vi "visitCompoundGraphic.vi"(8 "error in (no error)":errorcluster, 10 "CompoundShape":refnum<class "CompoundShape.lvclass">, 11 "XMLExportVisitor in":refnum<class "XMLExportVisitor.lvclass">) -> (0 "error out":errorcluster, 2 "String":string, 3 "XMLExportVisitor out":refnum<class "XMLExportVisitor.lvclass">)   [LabVIEW 2017, in "XMLExportVisitor.lvclass"]
uses:
  XMLExportVisitor.lvclass
  CompoundShape Class/CompoundShape.lvclass
  CompoundShape Class/CompoundShape.lvclass/CompoundShape.ctl
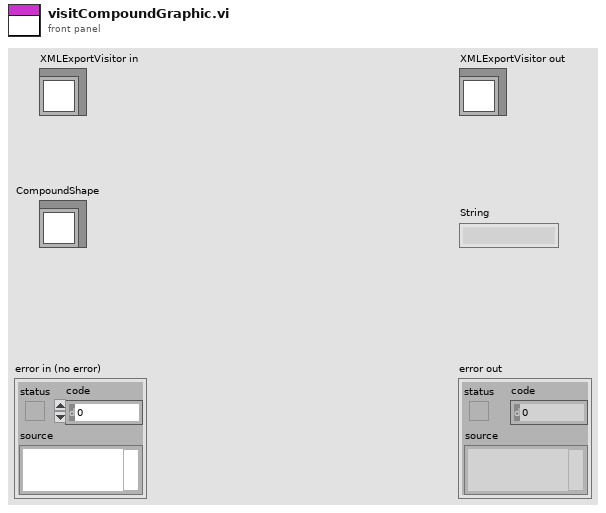
[diagram p1: front panel]
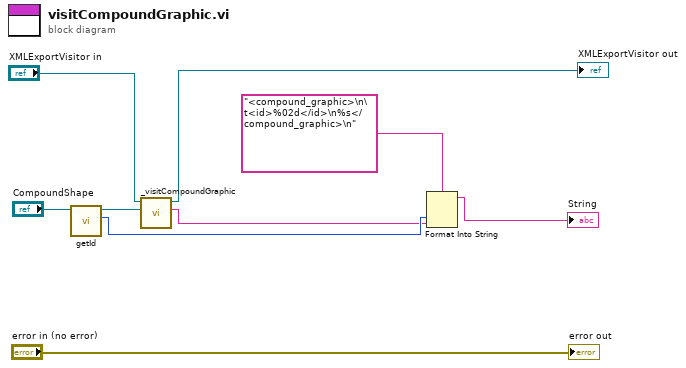
[diagram p0: block diagram]
diagram:
  n1 = call "getId.vi"("CompoundShape in"="CompoundShape") -> ("id"=w3:i32, "CompoundShape out"=w4:refnum<class "CompoundShape.lvclass">)  [unwired: 8 in, 1 out]
  n2 = call "_visitCompoundGraphic.vi"("CompoundShape"=w4, "XMLExportVisitor in"="XMLExportVisitor in") -> ("String"=w2:string, "XMLExportVisitor out"=→"XMLExportVisitor out":refnum<class "XMLExportVisitor.lvclass">)  [unwired: 7 in, 1 out]
  n3 = Format Into String(format string="<compound_graphic>\n\t<id>%02d</id>\n%s</compound_graphic>\n", w3, w2) -> (resulting string=→"String":string)  [unwired: 2 in, 1 out]
  "error out" <- "error in (no error)"
